vi "Select_Offset.vi"() -> (0 "Boolean 4":bool, 1 "Boolean 3":bool, 2 "Boolean 2":bool, 3 "Boolean":bool, 4 "Boolean 5":bool)   [LabVIEW 2015]
uses:
  Variables_Offset.vi
panel:
  in  "stop":bool
  out "valor 5":dbl
  out "valor 4":dbl
  out "valor 3":dbl
  out "valor 2":dbl
  out "valor 1":dbl
  in  "lvdtvol":bool
  in  "precamara":bool
  in  "lvdtaxial":bool
  in  "CCArga":bool
  in  "presporo":bool
  # "Offset"
  # "Sensor"
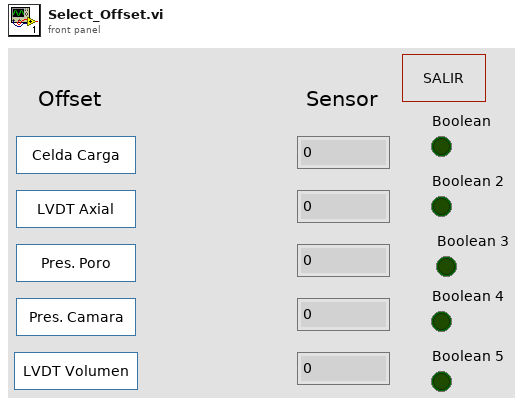
[diagram p1: front panel]
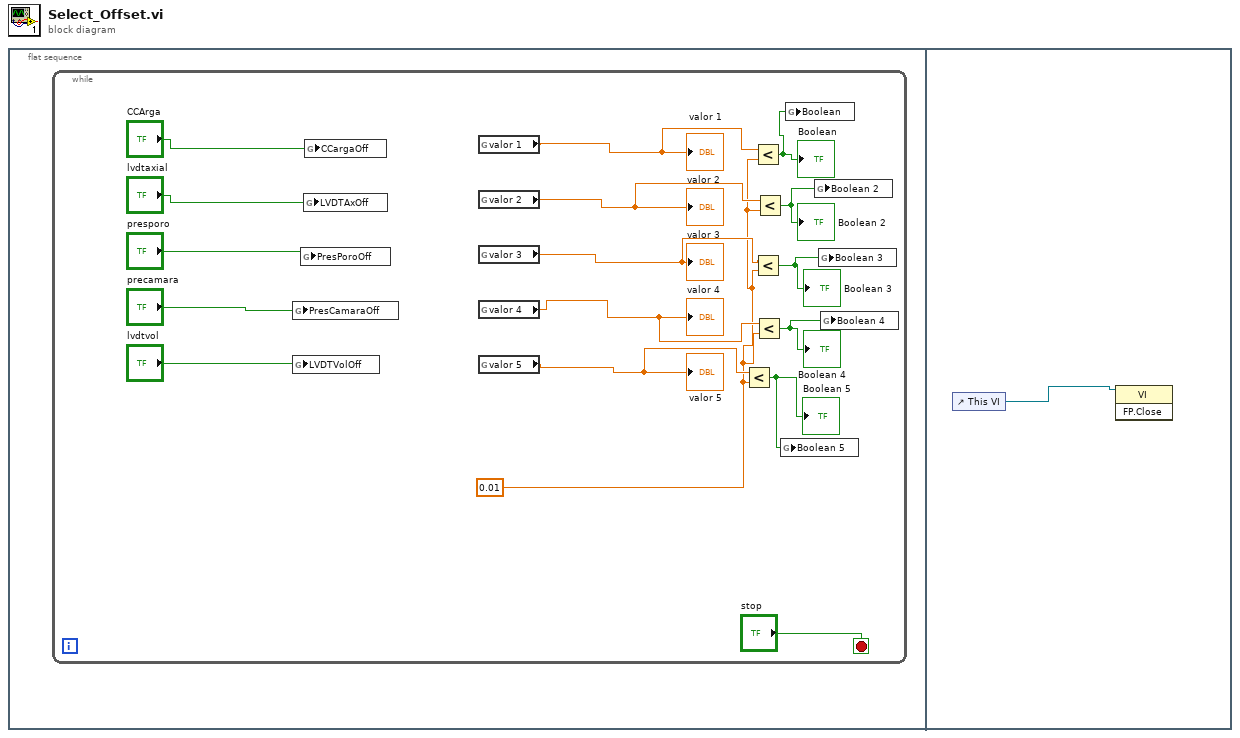
[diagram p0: block diagram]
diagram:
  n1 = flat-sequence {
    frame #0 {
      n2 = while {
        stop <- "stop" stop-if-true
        w6 = 0.01
        n3 = global write "Variables_Offset.vi" "PresCamaraOff"("precamara") -> ()
        n4 = global write "Variables_Offset.vi" "LVDTVolOff"("lvdtvol") -> ()
        n5 = global write "Variables_Offset.vi" "PresPoroOff"("presporo") -> ()
        n6 = global write "Variables_Offset.vi" "LVDTAxOff"("lvdtaxial") -> ()
        n7 = global write "Variables_Offset.vi" "CCargaOff"("CCArga") -> ()
        n8 = global read "Variables_Offset.vi" "valor 1"() -> (w7:dbl)
        "valor 1" <- w7
        n9 = global read "Variables_Offset.vi" "valor 2"() -> (w8:dbl)
        "valor 2" <- w8
        n10 = global read "Variables_Offset.vi" "valor 3"() -> (w9:dbl)
        "valor 3" <- w9
        n11 = global read "Variables_Offset.vi" "valor 4"() -> (w10:dbl)
        "valor 4" <- w10
        n12 = global read "Variables_Offset.vi" "valor 5"() -> (w11:dbl)
        "valor 5" <- w11
        n13 = Less?(x=w11, y=w6) -> (x < y?=w1:bool)
        "Boolean 5" <- w1
        n14 = Less?(x=w7, y=w6) -> (x < y?=w5:bool)
        "Boolean" <- w5
        n15 = Less?(x=w9, y=w6) -> (x < y?=w3:bool)
        "Boolean 3" <- w3
        n16 = Less?(x=w10, y=w6) -> (x < y?=w2:bool)
        "Boolean 4" <- w2
        n17 = Less?(x=w8, y=w6) -> (x < y?=w4:bool)
        "Boolean 2" <- w4
        n18 = global write "Variables_Offset.vi" "Boolean 5"(w1) -> ()
        n19 = global write "Variables_Offset.vi" "Boolean"(w5) -> ()
        n20 = global write "Variables_Offset.vi" "Boolean 2"(w4) -> ()
        n21 = global write "Variables_Offset.vi" "Boolean 3"(w3) -> ()
        n22 = global write "Variables_Offset.vi" "Boolean 4"(w2) -> ()
      }
    }
    frame #1 {
      n23 = control-ref of="This VI"() -> (w18:refnum<vi>)
      n24 = invoke class="VI" method="FP.Close"(reference=w18) -> ()  [unwired: 2 in, 3 out]
    }
  }
